vi "Joint_Command_Mode.vi"(0 "Side":T1, 1 "node":string, 2 "Mode":u8(ring) items=["Position", "Velocity", "Effort"], 3 "error in":errorcluster) -> (6 "error out":errorcluster)   [LabVIEW 2013]
uses:
  ROS/Code/SubVIs/BaxterSide.ctl
  ROS/MessageBuilding/Primitives/subs/u8Scalar.vi
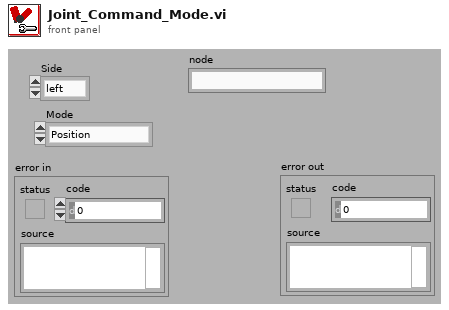
[diagram p1: front panel]
types:
  T1 = typedef "BaxterSide.ctl" = enum16{"left", "right"}
  T2 = typedef "_ROSControl.ctl" = cluster{"topic port":u16, "Node":string, "topic":string, "type":string, "node port":u32, "error ":errorcluster, "Direction":T3, "APIs":string[]}
  T3 = typedef "_ROSDirection.ctl" = enum16{"Node", "Publisher", "Subscriber", "Service Client"}
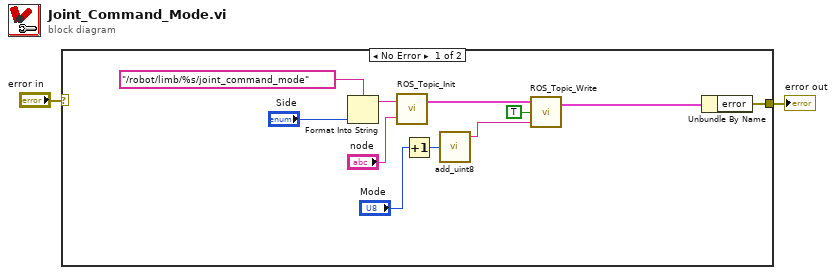
[diagram p0: block diagram]
diagram:
  n1 = case shown="No Error" "error in" {
    selector: "error in" -> [_ w14]
    tunnel: [w11 w14] -> w2
    frame No Error {
      n2 = Format Into String(format string="/robot/limb/%s/joint_command_mode" ("topic"), "Side") -> (resulting string=w8:string)  [unwired: 2 in, 1 out]
      n3 = call "ROS_Topic_Init.vi"("node"="node", "topic"=w8) -> ("ROS out"=w13:T2)  [unwired: 1 in]
      n4 = Increment(x="Mode") -> (x+1=w6:u8)
      n5 = call-poly "add_uint8.vi"("Numeric"=w6) -> ("msg out"=w5:string)  [unwired: 4 in]
      n6 = call "ROS_Topic_Write.vi"("Msg in"=w5, "Continuous?"=TRUE, "ROS in"=w13) -> ("ROS out"=w12:T2)  [unwired: 1 in]
      n7 = Unbundle By Name(w12) -> ("error"=w11:errorcluster)
    }
    frame Error {
    }
  }
  "error out" <- w2
